vi "Read-Write Python Version.vi"(7 "Version":string, 10 "Task":enum16{"Read", "Write"}(ring)) -> ()   [LabVIEW 2019]
uses:
  <userlib>/MicroPython/VIs/SSH/PythonVersion.vi
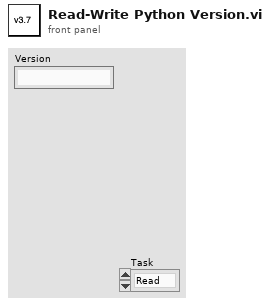
[diagram p1: front panel]
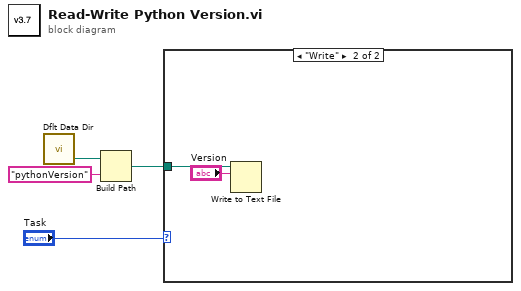
[diagram p0: block diagram]
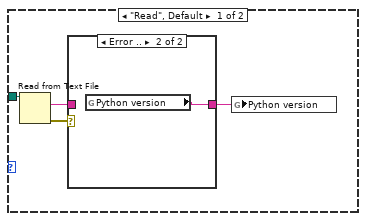
[diagram p2: hidden frame]
diagram:
  n1 = call <vilib>:"Dflt Data Dir.vi"() -> ("App:Default Data Directory"=w4:path)
  n2 = Build Path(base path=w4, name or relative path="pythonVersion") -> (appended path=w2:path)
  n3 = case shown="\"Write\"" "Task" {
    tunnel: w2 -> [w8 w12]
    frame "Read", Default {
      n4 = Read from Text File(file (use dialog)=w8) -> (text=w6:string, error out=w7:errorcluster)  [unwired: 3 in, 2 out]
      n5 = case shown="Error .." w7 {
        tunnel: [w9 w10] -> w5
        tunnel: w6 -> [w9 _]
        frame No Error {
        }
        frame Error {
          n6 = global read "PythonVersion.vi" "Python version"() -> (w10:string)
        }
      }
      n7 = global write "PythonVersion.vi" "Python version"(w5) -> ()
    }
    frame "Write" {
      n8 = Write to Text File(file (use dialog)=w12, text="Version") -> ()  [unwired: 2 in, 3 out]
    }
  }
